vi "Initialization VI.vi"(8 "error in (no error)":errorcluster, 10 "Custom XML":string, 11 "Device Item Ref in":T1 format="%.0x") -> (0 "error out":errorcluster, 3 "Device Item Ref out":T1 format="%.0x")   [LabVIEW 2021, in "G5 Regatron Custom Device System Explorer.lvlib"]
uses:
  G5 Regatron Custom Device System Explorer.lvlib
  <vilib>/NI VeriStand/Custom Device API/Custom Device Item Ref.ctl
  <vilib>/NI VeriStand/Custom Device API/Custom Device Channel.ctl
  <vilib>/NI VeriStand/Custom Device API/Custom Device Channel Type.ctl
  <vilib>/NI/NI VeriStand Custom Device Import and Export Tool/ImportExport.lvlib
  <vilib>/NI VeriStand/Custom Device API/Custom Device API.lvlib
  <vilib>/NI VeriStand/Custom Device API/Custom Device Loop Type.ctl
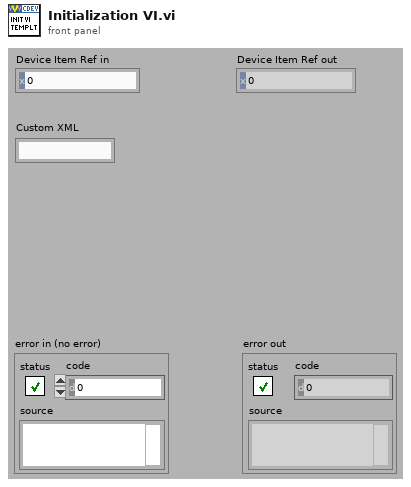
[diagram p1: front panel]
types:
  T1 = typedef "Custom Device API.lvlib/Custom Device Item Ref.ctl" = u64
  T2 = typedef "Custom Device API.lvlib/Custom Device Loop Type.ctl" = enum32{"While Loop", "Timed Loop"}
  T3 = typedef "Custom Device API.lvlib/Custom Device Channel.ctl" = cluster{"Type":T4, "Units":string, "Default Value":dbl, "Faultable":bool, "Scalable":bool}
  T4 = typedef "Custom Device API.lvlib/Custom Device Channel Type.ctl" = enum16{"Input", "Output"}
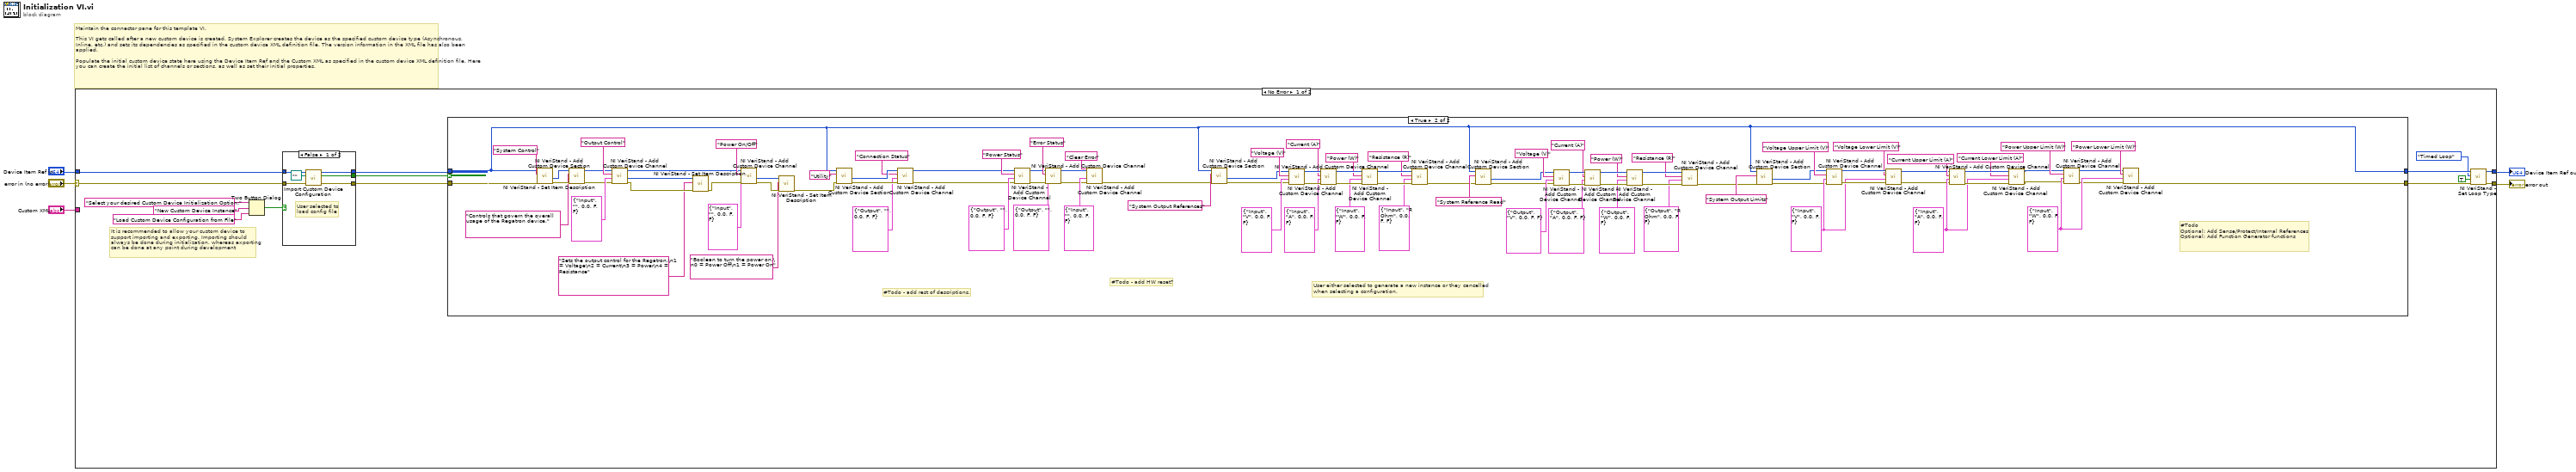
[diagram p0: block diagram]
diagram:
  # "Maintain the connector pane for this template VI.\n\nThis VI gets called after a new custom device is created. System Explorer creates the device as the specified custom device type (Asynchronous, Inline, etc.) and sets its dependencies as specified in the custom device XML definition file. The version information in the XML file has also been applied.\n\nPopulate the initial custom device state here using the Device Item Ref and the Custom XML as specified in the custom device XML definition file. Here you can create the initial list of channels or sections, as well as set their initial properties."
  n1 = case shown="No Error" "error in (no error)" {
    selector: "error in (no error)" -> [w15 w131]
    tunnel: [w8 w131] -> w5
    tunnel: [w10 w130] -> w3
    tunnel: "Device Item Ref in" -> [w16 w130]
    tunnel: "Custom XML" -> [_ _]
    frame No Error {
      # "It is recommended to allow your custom device to\nsupport importing and exporting. Importing should\nalways be done during initialization, whereas exporting\ncan be done at any point during development"
      n2 = Two Button Dialog(message="Select your desired Custom Device Initialization Option:", 1:"Load Custom Device Configuration from File" ("F button name (\"Cancel\")"), 2:"New Custom Device Instance" ("T button name (\"OK\")")) -> (T button?=w17:bool)
      n3 = case shown="False" w17 {
        selector: w17 -> [_ w127]
        tunnel: w16 -> [w126 w129]
        tunnel: [w125 w129] -> w14
        tunnel: w15 -> [w123 w128]
        tunnel: [w122 w128] -> w12
        tunnel: [w121 w127] -> w13
        frame False {
          # "User selected to\nload config file"
          n4 = call <vilib>:"Import Custom Device Configuration.vi"("error in (no error)"=w123, "Path"=path "", "NodeID"=w126) -> ("error out"=w122:errorcluster, "cancelled"=w121:bool, "NodeID out"=w125:u64)  [unwired: 6 in]
        }
        frame True {
          # "User selected new\ncustom device. Do\nnothing in this case\nand handle new\ngeneration in the\nnext case structure"
        }
      }
      n5 = case shown="True" w13 {
        tunnel: w14 -> [w22 w37]
        tunnel: w12 -> [w21 w96]
        tunnel: [w21 w36] -> w9
        tunnel: [w22 w37] -> w11
        frame False {
          # "User selected to import from configuration and didn't cancel import"
        }
        frame True {
          w44 = T3 {"Type"=enum."Input", "Units"="W", "Default Value"=0.0, "Faultable"=FALSE, "Scalable"=FALSE} ("Channel")
          w49 = T3 {"Type"=enum."Input", "Units"="V", "Default Value"=0.0, "Faultable"=FALSE, "Scalable"=FALSE} ("Channel")
          w107 = T3 {"Type"=enum."Input", "Units"="A", "Default Value"=0.0, "Faultable"=FALSE, "Scalable"=FALSE} ("Channel")
          # "#Todo - add rest of descriptions."
          # "#Todo - add HW reset?"
          # "#Todo\nOptional: Add Sense/Protect/Internal References\nOptional: Add Function Generator functions"
          # "User either selected to generate a new instance or they cancelled\nwhen selecting a configuration."
          n6 = call <vilib>:"NI VeriStand - Add Custom Device Section.vi"("error in (no error)"=w96, "Section Name"="System Control", "Parent Ref in"=w37) -> ("error out"=w27:errorcluster, "Section Ptr"=w25:T1)  [unwired: 5 in, 2 out]
          n7 = call <vilib>:"NI VeriStand - Set Item Description.vi"("error in (no error)"=w27, "Description"="Controls that govern the overall usage of the Regatron device.", "Item Ref in"=w25) -> ("error out"=w26:errorcluster, "Item Ref out"=w24:T1)  [unwired: 6 in, 1 out]
          n8 = call <vilib>:"NI VeriStand - Add Custom Device Channel.vi"("error in (no error)"=w26, "Channel"=T3 {"Type"=enum."Input", "Units"="", "Default Value"=0.0, "Faultable"=FALSE, "Scalable"=FALSE}, "Channel Name"="Output Control", "Parent Ref in"=w24) -> ("error out"=w34:errorcluster, "Channel Ref"=w35:T1, "Parent Ref out"=w94:T1)  [unwired: 4 in, 1 out]
          n9 = call <vilib>:"NI VeriStand - Set Item Description.vi"("error in (no error)"=w34, "Description"="Sets the output control for the Regatron.\n1 = Voltage\n2 = Current\n3 = Power\n4 = Resistance", "Item Ref in"=w35) -> ("error out"=w33:errorcluster)  [unwired: 6 in, 2 out]
          n10 = call <vilib>:"NI VeriStand - Add Custom Device Channel.vi"("error in (no error)"=w33, "Channel"=T3 {"Type"=enum."Input", "Units"="", "Default Value"=0.0, "Faultable"=FALSE, "Scalable"=FALSE}, "Channel Name"="Power On/Off", "Parent Ref in"=w94) -> ("error out"=w31:errorcluster, "Channel Ref"=w29:T1)  [unwired: 4 in, 2 out]
          n11 = call <vilib>:"NI VeriStand - Set Item Description.vi"("error in (no error)"=w31, "Description"="Boolean to turn the power on.\n0 = Power Off\n1 = Power On", "Item Ref in"=w29) -> ("error out"=w30:errorcluster)  [unwired: 6 in, 2 out]
          n12 = call <vilib>:"NI VeriStand - Add Custom Device Section.vi"("error in (no error)"=w30, "Section Name"="Utility", "Parent Ref in"=w37) -> ("error out"=w84:errorcluster, "Section Ptr"=w81:T1)  [unwired: 5 in, 2 out]
          n13 = call <vilib>:"NI VeriStand - Add Custom Device Channel.vi"("error in (no error)"=w84, "Channel"=T3 {"Type"=enum."Output", "Units"="", "Default Value"=0.0, "Faultable"=FALSE, "Scalable"=FALSE}, "Channel Name"="Connection Status", "Parent Ref in"=w81) -> ("error out"=w82:errorcluster, "Parent Ref out"=w80:T1)  [unwired: 4 in, 2 out]
          n14 = call <vilib>:"NI VeriStand - Add Custom Device Channel.vi"("error in (no error)"=w82, "Channel"=T3 {"Type"=enum."Output", "Units"="", "Default Value"=0.0, "Faultable"=FALSE, "Scalable"=FALSE}, "Channel Name"="Power Status", "Parent Ref in"=w80) -> ("error out"=w91:errorcluster, "Parent Ref out"=w93:T1)  [unwired: 4 in, 2 out]
          n15 = call <vilib>:"NI VeriStand - Add Custom Device Channel.vi"("error in (no error)"=w91, "Channel"=T3 {"Type"=enum."Output", "Units"="", "Default Value"=0.0, "Faultable"=FALSE, "Scalable"=FALSE}, "Channel Name"="Error Status", "Parent Ref in"=w93) -> ("error out"=w90:errorcluster, "Parent Ref out"=w92:T1)  [unwired: 4 in, 2 out]
          n16 = call <vilib>:"NI VeriStand - Add Custom Device Channel.vi"("error in (no error)"=w90, "Channel"=T3 {"Type"=enum."Input", "Units"="", "Default Value"=0.0, "Faultable"=FALSE, "Scalable"=FALSE}, "Channel Name"="Clear Error", "Parent Ref in"=w92) -> ("error out"=w85:errorcluster)  [unwired: 4 in, 3 out]
          n17 = call <vilib>:"NI VeriStand - Add Custom Device Section.vi"("error in (no error)"=w85, "Section Name"="System Output References", "Parent Ref in"=w37) -> ("error out"=w87:errorcluster, "Section Ptr"=w88:T1)  [unwired: 5 in, 2 out]
          n18 = call <vilib>:"NI VeriStand - Add Custom Device Channel.vi"("error in (no error)"=w87, "Channel"=T3 {"Type"=enum."Input", "Units"="V", "Default Value"=0.0, "Faultable"=FALSE, "Scalable"=FALSE}, "Channel Name"="Voltage (V)", "Parent Ref in"=w88) -> ("error out"=w118:errorcluster, "Parent Ref out"=w117:T1)  [unwired: 4 in, 2 out]
          n19 = call <vilib>:"NI VeriStand - Add Custom Device Channel.vi"("error in (no error)"=w118, "Channel"=T3 {"Type"=enum."Input", "Units"="A", "Default Value"=0.0, "Faultable"=FALSE, "Scalable"=FALSE}, "Channel Name"="Current (A)", "Parent Ref in"=w117) -> ("error out"=w116:errorcluster, "Parent Ref out"=w115:T1)  [unwired: 4 in, 2 out]
          n20 = call <vilib>:"NI VeriStand - Add Custom Device Channel.vi"("error in (no error)"=w116, "Channel"=T3 {"Type"=enum."Input", "Units"="W", "Default Value"=0.0, "Faultable"=FALSE, "Scalable"=FALSE}, "Channel Name"="Power (W)", "Parent Ref in"=w115) -> ("error out"=w113:errorcluster, "Parent Ref out"=w112:T1)  [unwired: 4 in, 2 out]
          n21 = call <vilib>:"NI VeriStand - Add Custom Device Channel.vi"("error in (no error)"=w113, "Channel"=T3 {"Type"=enum."Input", "Units"="R Ohm", "Default Value"=0.0, "Faultable"=FALSE, "Scalable"=FALSE}, "Channel Name"="Resistance (R)", "Parent Ref in"=w112) -> ("error out"=w55:errorcluster)  [unwired: 4 in, 3 out]
          n22 = call <vilib>:"NI VeriStand - Add Custom Device Section.vi"("error in (no error)"=w55, "Section Name"="System Reference Read", "Parent Ref in"=w37) -> ("error out"=w61:errorcluster, "Section Ptr"=w62:T1)  [unwired: 5 in, 2 out]
          n23 = call <vilib>:"NI VeriStand - Add Custom Device Channel.vi"("error in (no error)"=w61, "Channel"=T3 {"Type"=enum."Output", "Units"="V", "Default Value"=0.0, "Faultable"=FALSE, "Scalable"=FALSE}, "Channel Name"="Voltage (V)", "Parent Ref in"=w62) -> ("error out"=w70:errorcluster, "Parent Ref out"=w69:T1)  [unwired: 4 in, 2 out]
          n24 = call <vilib>:"NI VeriStand - Add Custom Device Channel.vi"("error in (no error)"=w70, "Channel"=T3 {"Type"=enum."Output", "Units"="A", "Default Value"=0.0, "Faultable"=FALSE, "Scalable"=FALSE}, "Channel Name"="Current (A)", "Parent Ref in"=w69) -> ("error out"=w68:errorcluster, "Parent Ref out"=w67:T1)  [unwired: 4 in, 2 out]
          n25 = call <vilib>:"NI VeriStand - Add Custom Device Channel.vi"("error in (no error)"=w68, "Channel"=T3 {"Type"=enum."Output", "Units"="W", "Default Value"=0.0, "Faultable"=FALSE, "Scalable"=FALSE}, "Channel Name"="Power (W)", "Parent Ref in"=w67) -> ("error out"=w65:errorcluster, "Parent Ref out"=w64:T1)  [unwired: 4 in, 2 out]
          n26 = call <vilib>:"NI VeriStand - Add Custom Device Channel.vi"("error in (no error)"=w65, "Channel"=T3 {"Type"=enum."Output", "Units"="R Ohm", "Default Value"=0.0, "Faultable"=FALSE, "Scalable"=FALSE}, "Channel Name"="Resistance (R)", "Parent Ref in"=w64) -> ("error out"=w54:errorcluster)  [unwired: 4 in, 3 out]
          n27 = call <vilib>:"NI VeriStand - Add Custom Device Section.vi"("error in (no error)"=w54, "Section Name"="System Output Limits", "Parent Ref in"=w37) -> ("error out"=w48:errorcluster, "Section Ptr"=w47:T1)  [unwired: 5 in, 2 out]
          n28 = call <vilib>:"NI VeriStand - Add Custom Device Channel.vi"("error in (no error)"=w48, "Channel"=w49, "Channel Name"="Voltage Upper Limit (V)", "Parent Ref in"=w47) -> ("error out"=w52:errorcluster, "Parent Ref out"=w51:T1)  [unwired: 4 in, 2 out]
          n29 = call <vilib>:"NI VeriStand - Add Custom Device Channel.vi"("error in (no error)"=w52, "Channel"=w49, "Channel Name"="Voltage Lower Limit (V)", "Parent Ref in"=w51) -> ("error out"=w45:errorcluster, "Parent Ref out"=w46:T1)  [unwired: 4 in, 2 out]
          n30 = call <vilib>:"NI VeriStand - Add Custom Device Channel.vi"("error in (no error)"=w45, "Channel"=w107, "Channel Name"="Current Upper Limit (A)", "Parent Ref in"=w46) -> ("error out"=w110:errorcluster, "Parent Ref out"=w109:T1)  [unwired: 4 in, 2 out]
          n31 = call <vilib>:"NI VeriStand - Add Custom Device Channel.vi"("error in (no error)"=w110, "Channel"=w107, "Channel Name"="Current Lower Limit (A)", "Parent Ref in"=w109) -> ("error out"=w38:errorcluster, "Parent Ref out"=w39:T1)  [unwired: 4 in, 2 out]
          n32 = call <vilib>:"NI VeriStand - Add Custom Device Channel.vi"("error in (no error)"=w38, "Channel"=w44, "Channel Name"="Power Upper Limit (W)", "Parent Ref in"=w39) -> ("error out"=w41:errorcluster, "Parent Ref out"=w42:T1)  [unwired: 4 in, 2 out]
          n33 = call <vilib>:"NI VeriStand - Add Custom Device Channel.vi"("error in (no error)"=w41, "Channel"=w44, "Channel Name"="Power Lower Limit (W)", "Parent Ref in"=w42) -> ("error out"=w36:errorcluster)  [unwired: 4 in, 3 out]
        }
      }
      n34 = call <vilib>:"NI VeriStand - Set Loop Type.vi"("error in (no error)"=w9, "Use Device Clock (Timed Loops only)"=TRUE, "Loop type"=Custom_Device_Loop_Type."Timed Loop", "Device Ref in"=w11) -> ("error out"=w8:errorcluster, "Device Ref out"=w10:T1)  [unwired: 6 in]
    }
    frame Error {
    }
  }
  "error out" <- w5
  "Device Item Ref out" <- w3
